vi "Test Test Finder Find Static Test Methods in Test Case Class.vi"(8 "error in (no error)":errorcluster, 11 "Test Finder In":refnum<class "Test Finder.lvclass">) -> (0 "error out":errorcluster, 3 "Test Finder Out":refnum<class "Test Finder.lvclass">)   [LabVIEW 2020, in "LUnit Tests.lvlib" / "Test Finder.lvclass"]
uses:
  Test Finder.lvclass
  Test Dummys/Descending Test Test Case/Descending Test Test Case.lvclass
  Test Finder.lvclass/Test Finder.ctl
  <vilib>/Astemes/LUnit/Test Case.lvclass/Test Case.ctl
  <vilib>/Astemes/LUnit/LUnit Assertion Result.lvclass/LUnit Assertion Result.ctl
  <vilib>/Astemes/LUnit/LUnit Test Case Result.lvclass/LUnit Test Case Result.ctl
  <vilib>/Astemes/LUnit/LUnit Method Result.lvclass/LUnit Method Result.ctl
  <vilib>/Astemes/LUnit/Palette/Fail.vi
  <vilib>/Astemes/LUnit/Palette/Pass.vi
  <vilib>/Astemes/LUnit/Set Assertion Type.vi
  <vilib>/Astemes/LUnit/Add test result.vi
  <vilib>/Astemes/LUnit/LUnit Write Passed.vi
  <vilib>/Astemes/LUnit/LUnit Write Message.vi
  <vilib>/Astemes/LUnit/LUnit Write Description.vi
  <vilib>/Astemes/LUnit/LUnit Write Assertion Type.vi
  <vilib>/Astemes/LUnit/LUnit Record Assertion Result.vi
  <vilib>/Astemes/LUnit/LUnit Aggregate Assertion Results.vi
  <vilib>/Astemes/LUnit/Assertion Result/LUnit Read Status.vi
  <vilib>/Astemes/LUnit/LUnit Read Message.vi
  <vilib>/Astemes/LUnit/LUnit Read Description.vi
  <vilib>/Astemes/LUnit/Method Result/LUnit Merge Status.vi
  <vilib>/Astemes/LUnit/LUnit Concatenate result strings.vi
  source/Framework/Helper Classes/Test Finder/Test Finder.lvclass
  <vilib>/Astemes/LUnit/LUnit Assertion Result.lvclass
  32a5955b-25e4-4671-b4b3-9f259fd0ce92.vi
  C:/Git/astemes-lunit/tests/Test Dummys/Test Test Case/Test Test Case.lvclass
  C:/Git/astemes-lunit/source/Framework/Test Case/LUnit Test Case.lvclass
  C:/Git/astemes-lunit/tests/Test Dummys/Descending Test Test Case/Descending Test Test Case.lvclass
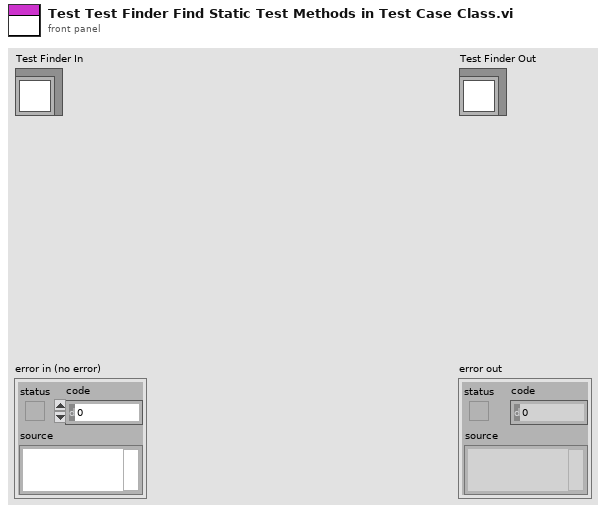
[diagram p1: front panel]
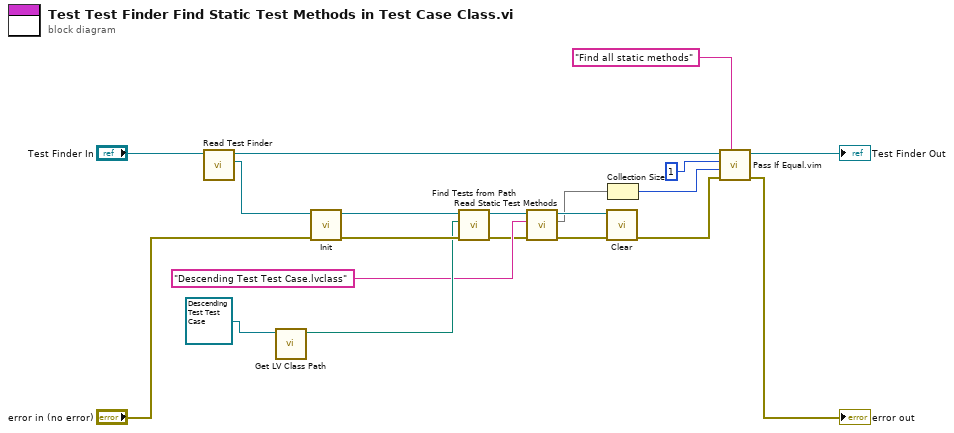
[diagram p0: block diagram]
diagram:
  n1 = call "Read Test Finder.vi"("Test Finder In"="Test Finder In") -> ("Test Finder.lvclass"=w19:refnum<class "Test Finder.lvclass">, "Test Finder Out"=w8:refnum<class "Test Finder.lvclass">)  [unwired: 8 in, 1 out]
  n2 = call <vilib>:"Get LV Class Path.vi"("object"=refnum<class "Descending Test Test Case.lvclass"> refnum ("Descending Test Test Case.lvclass")) -> ("class path"=w15:path)  [unwired: 9 in, 1 out]
  n3 = call-dynamic "Init.vi"("error in (no error)"="error in (no error)", "Test Finder in"=w19) -> ("error out"=w17:errorcluster, "Test Finder out"=w18:refnum<class "Test Finder.lvclass">)  [unwired: 8 in]
  n4 = call-dynamic "Find Tests from Path.vi"("error in (no error)"=w17, "Project or Class Path"=w15, "Test Case Finder In"=w18) -> ("error out"=w11:errorcluster, "Test Case Finder Out"=w13:refnum<class "Test Finder.lvclass">)  [unwired: 7 in]
  n5 = call "Read Static Test Methods.vi"("error in (no error)"=w11, "Test Case"="Descending Test Test Case.lvclass", "Test Case Finder In"=w13) -> ("error out"=w10:errorcluster, "Static Test Methods"=w4:map{string, path}, "Test Case Finder Out"=w12:refnum<class "Test Finder.lvclass">)  [unwired: 6 in]
  n6 = call "Clear.vi"("error in (no error)"=w10, "Test Finder in"=w12) -> ("error out"=w6:errorcluster)  [unwired: 8 in, 1 out]
  n7 = Collection Size(1:w4) -> (0:w2:i32)
  n8 = call "Pass If Equal.vim"("Description"="Find all static methods", "error in (no error)"=w6, "Actual"=w2, "Expected"=1 ("size"), "LUnit Test Case In"=w8) -> ("error out"=→"error out":errorcluster, "LUnit Test Case Out"=→"Test Finder Out":refnum<class "Test Finder.lvclass">)  [unwired: 5 in]
